vi "Autonomous Independent.vi"() -> ()   [LabVIEW 2014]
doc: "This VI is called when autonomous begins, and will automatically be terminated when autonomous ends. You can carry out timed or sensor driven robot movement independently without needing to return to the caller."
uses:
  <vilib>/Rock Robotics/Network Tables/SD Read String.vi
  Robot Global Data.vi
panel:
  out "Angular Target":dbl(graph)
  out "Y Values":dbl(graph)
  out "X Values":dbl(graph)
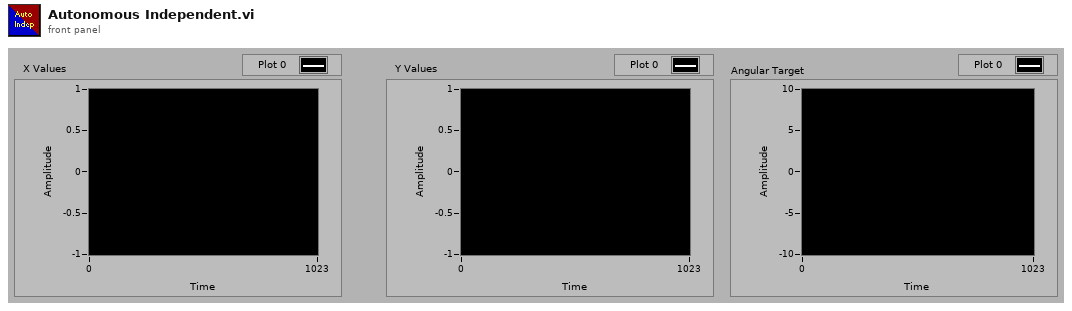
[diagram p1: front panel]
types:
  T1 = cluster{dbl[], dbl[], dbl[], dbl[], dbl[], dbl[], dbl[], dbl[], dbl[]}
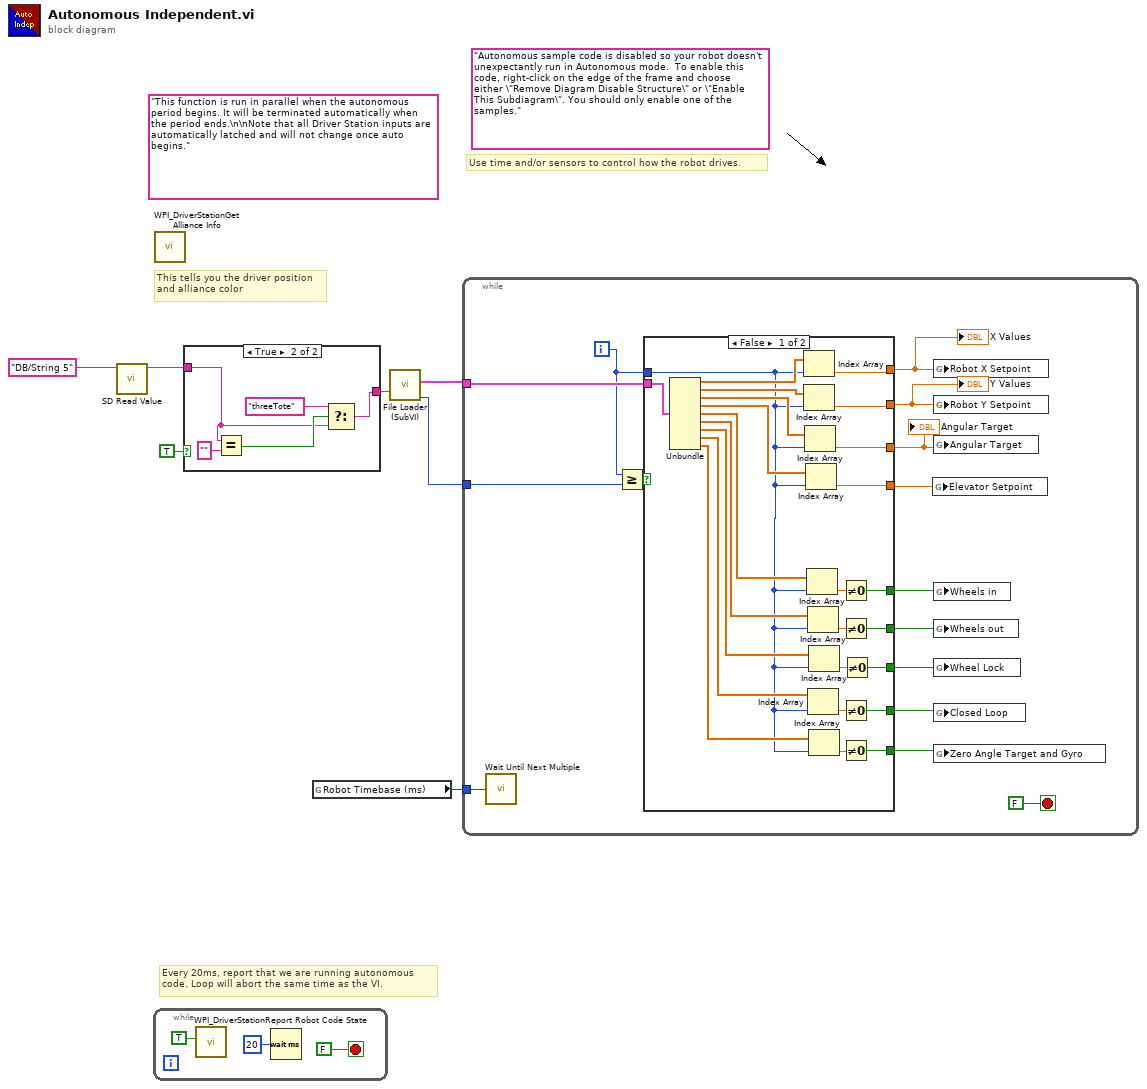
[diagram p0: block diagram]
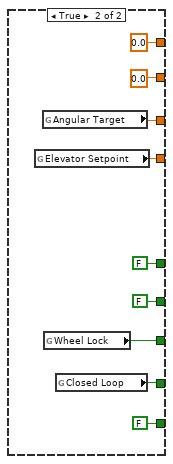
[diagram p3: hidden frame]
diagram:
  (unwired) "Autonomous sample code is disabled so your robot doesn't unexpectantly run in Autonomous mode.  To enable this code, right-click on the edge of the frame and choose either \"Remove Diagram Disable Structure\" or \"Enable This Subdiagram\". You should only enable one of the samples."
  (unwired) "This function is run in parallel when the autonomous period begins. It will be terminated automatically when the period ends.\n\nNote that all Driver Station inputs are automatically latched and will not change once auto begins."
  # "Every 20ms, report that we are running autonomous\ncode. Loop will abort the same time as the VI."
  # "Use time and/or sensors to control how the robot drives."
  # "This tells you the driver position\nand alliance color"
  n1 = call-poly <vilib>:"SD Read Value.vi"("Name"="DB/String 5") -> ("String"=w3:string)  [unwired: 8 in, 2 out]
  n2 = while {
    stop <- FALSE stop-if-true
    n3 = call <vilib>:"WPI_DriverStationReport Robot Code State.vi"("Autonomous"=TRUE) -> ()  [unwired: 10 in, 1 out]
    n4 = Wait (ms)(milliseconds to wait=u32 20) -> ()  [unwired: 1 out]
  }
  n5 = call <vilib>:"WPI_DriverStationGet Alliance Info.vi"() -> ()  [unwired: 12 out]
  n6 = case shown="True" TRUE {
    tunnel: w3 -> [w11 w13]
    tunnel: [w11 w12] -> w2
    frame False {
    }
    frame True {
      n7 = Equal?(x=w13, y="") -> (x = y?=w15:bool)
      n8 = Select(t="threeTote", s=w15, f=w13) -> (s? t:f=w12:string)
    }
  }
  n9 = global read "Robot Global Data.vi" "Robot Timebase (ms)"() -> (w6:u32)
  n10 = call "File Loader (SubVI).vi"("Filename In"=w2) -> ("Number of Records"=w7:i32, "output cluster"=w5:T1)  [unwired: 6 in, 1 out]
  n11 = while {
    tunnel: w5 -> [w31]
    tunnel: w7 -> [w29]
    tunnel: w6 -> [w26]
    i -> [w30]
    stop <- FALSE stop-if-true
    n12 = call "Wait Until Next Multiple"("Count(mSec)"=w26) -> ()  [unwired: 1 out]
    n13 = Greater Or Equal?(x=w30, y=w29) -> (x >= y?=w28:bool)
    n14 = case shown="False" w28 {
      tunnel: w31 -> [w56 _]
      tunnel: w30 -> [w32 _]
      tunnel: [w50 w65] -> w25
      tunnel: [w54 0.0 ("Robot X Setpoint")] -> w19
      tunnel: [w52 0.0 ("Robot Y Setpoint")] -> w18
      tunnel: [w48 w62] -> w24
      tunnel: [w43 FALSE] -> w23
      tunnel: [w42 FALSE] -> w22
      tunnel: [w41 w59] -> w21
      tunnel: [w40 FALSE] -> w20
      tunnel: [w35 w57] -> w17
      frame False {
        n15 = Unbundle(w56) -> (w55:dbl[], w53:dbl[], w51:dbl[], w49:dbl[], w39:dbl[], w38:dbl[], w33:dbl[], w36:dbl[], w37:dbl[])
        n16 = Index Array(array=w55, index=w32) -> (element=w54:dbl)
        n17 = Index Array(array=w53, index=w32) -> (element=w52:dbl)
        n18 = Index Array(array=w51, index=w32) -> (element=w50:dbl)
        n19 = Index Array(array=w49, index=w32) -> (element=w48:dbl)
        n20 = Index Array(array=w39, index=w32) -> (element=w47:dbl)
        n21 = Index Array(array=w38, index=w32) -> (element=w46:dbl)
        n22 = Index Array(array=w36, index=w32) -> (element=w45:dbl)
        n23 = Index Array(array=w33, index=w32) -> (element=w34:dbl)
        n24 = Index Array(array=w37, index=w32) -> (element=w44:dbl)
        n25 = Not Equal To 0?(x=w47) -> (x != 0?=w43:bool)
        n26 = Not Equal To 0?(x=w46) -> (x != 0?=w42:bool)
        n27 = Not Equal To 0?(x=w45) -> (x != 0?=w41:bool)
        n28 = Not Equal To 0?(x=w44) -> (x != 0?=w40:bool)
        n29 = Not Equal To 0?(x=w34) -> (x != 0?=w35:bool)
      }
      frame True {
        n30 = global read "Robot Global Data.vi" "Elevator Setpoint"() -> (w62:dbl)
        n31 = global read "Robot Global Data.vi" "Angular Target"() -> (w65:dbl)
        n32 = global read "Robot Global Data.vi" "Wheel Lock"() -> (w57:bool)
        n33 = global read "Robot Global Data.vi" "Closed Loop"() -> (w59:bool)
      }
    }
    "X Values" <- w19
    "Y Values" <- w18
    "Angular Target" <- w25
    n34 = global write "Robot Global Data.vi" "Elevator Setpoint"(w24) -> ()
    n35 = global write "Robot Global Data.vi" "Robot X Setpoint"(w19) -> ()
    n36 = global write "Robot Global Data.vi" "Robot Y Setpoint"(w18) -> ()
    n37 = global write "Robot Global Data.vi" "Angular Target"(w25) -> ()
    n38 = global write "Robot Global Data.vi" "Wheels in"(w23) -> ()
    n39 = global write "Robot Global Data.vi" "Wheels out"(w22) -> ()
    n40 = global write "Robot Global Data.vi" "Wheel Lock"(w17) -> ()
    n41 = global write "Robot Global Data.vi" "Closed Loop"(w21) -> ()
    n42 = global write "Robot Global Data.vi" "Zero Angle Target and Gyro"(w20) -> ()
  }
